vi "Local Transition Inward.vi"(8 "error in (no error)":errorcluster, 10 "Target State":refnum<class "State Machine.lvclass">, 11 "State Machine in":refnum<class "State Machine.lvclass">) -> (0 "error out":errorcluster, 3 "State Machine out":refnum<class "State Machine.lvclass">)   [LabVIEW 2024, in "State Pattern Actor.lvlib" / "State Machine.lvlib" / "State Machine.lvclass"]
uses:
  State Machine.lvclass
  State Machine.lvclass/State Machine.ctl
  <vilib>/ActorFramework/Actor/Actor.lvclass
  C:/Program Files (x86)/National Instruments/LabVIEW 2024/vi.lib/ActorFramework/Actor/Actor.lvclass
  C:/Users/uspoaotto/OneDrive - Oregon Tool/Desktop/working copies/stateMachineActor/src/State Pattern Actor/State Machine Actor/State Machine.lvclass
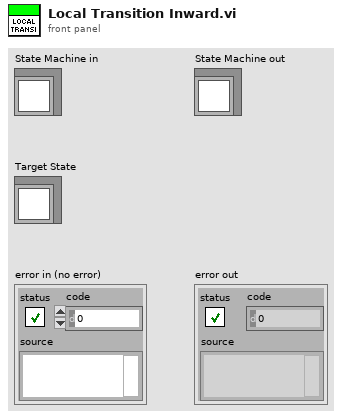
[diagram p1: front panel]
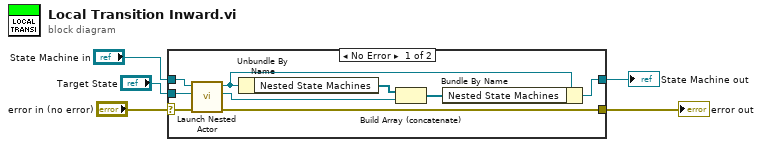
[diagram p0: block diagram]
diagram:
  n1 = case shown="No Error" "error in (no error)" {
    selector: "error in (no error)" -> [w11 w16]
    tunnel: [w10 w16] -> w4
    tunnel: [w9 w15] -> w2
    tunnel: "State Machine in" -> [w8 w15]
    tunnel: "Target State" -> [w7 _]
    frame No Error {
      n2 = call <vilib>:"Launch Nested Actor.vi"("error in (no error)"=w11, "Nested Actor"=w7, "Caller Actor in"=w8) -> ("error out"=w10:errorcluster, "Nested Actor's Enqueuer"=w13:refnum<class "Message Enqueuer.lvclass">, "Caller Actor out"=w6:refnum<class "State Machine.lvclass">)  [unwired: 6 in]
      n3 = Unbundle By Name(w6) -> ("Nested State Machines"=w14:refnum<class "Message Enqueuer.lvclass">[])
      n4 = Build Array (concatenate)(w14, w13) -> (w12:refnum<class "Message Enqueuer.lvclass">[])
      n5 = Bundle By Name(cluster=w6, "Nested State Machines"=w12) -> (w9:refnum<class "State Machine.lvclass">)
    }
    frame Error {
    }
  }
  "error out" <- w4
  "State Machine out" <- w2
